vi "RT Main - 9035.vi"() -> ()   [LabVIEW 2017]
uses:
  Controls/Logging Settings.ctl
  Support Vis/Message Queue/Message Cluster.ctl
  Controls/Manual Control.ctl
  Controls/Manual Control FPGA.ctl
  Controls/Logging Settings FPGA.ctl
  Globals/Host/Global - Configuration Options.vi
  Globals/RT/Globals - RT Stream.vi
  <vilib>/Utility/error.llb/Error Cluster From Error Code.vi
  <vilib>/rvi/errors/niLvFpgaAdjustHostInterfaceError.vi
  Globals/RT/Global - Valves.vi
  <vilib>/rvi/interface/nirviReadWriteControl/nirviReadWriteControl.xnode
  Support Vis/Message Queue/Message Queue.lvlib
  NiFpgaLv.dll
  <vilib>/rvi/interface/Simulation/niFpgaSimulationCallBeginRW.vi
panel:
  out "Ready to log":bool
  out "Logging Information":T1={"Logging Channels"={"TC Logging"={"TC 0"=FALSE, "TC 1"=FALSE, "TC 2"=FALSE, "TC 3"=FALSE, "TC 4"=FALSE, "TC 5"=FALSE, "TC 6"=FALSE, "TC 7"=FALSE, "TC 8"=FALSE, "TC 9"=FALSE, "TC 10"=FALSE, "TC 11"=FALSE, "TC 12"=FALSE, "TC 13"=FALSE, "TC 14"=FALSE, "TC 15"=FALSE}, "PS Logging"={"PS 0"=FALSE, "PS 1"=FALSE, "PS 2"=FALSE, "PS 3"=FALSE, "PS 4"=FALSE, "PS 5"=FALSE, "PS 6"=FALSE, "PS 7"=FALSE}, "LC Logging"={"LC 0"=FALSE, "LC 1"=FALSE, "LC 2"=FALSE, "LC 3"=FALSE}}, "TC Low Speed Logging [Hz]"=1, "TC High Speed Logging [Hz]"=1, "PS Low Speed Logging [Hz]"=1, "PS High Speed Logging [Hz]"=1, "LC Low Speed Logging [Hz]"=1, "LC High Speed Logging[Hz]"=1, "Valve Names"=[]}
  out "Logging":bool
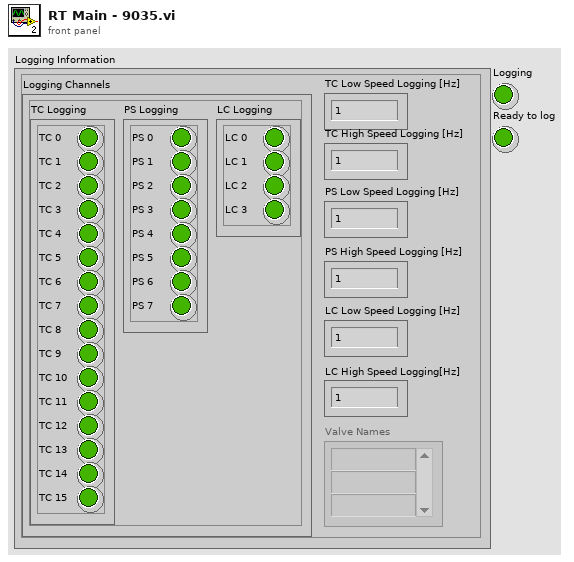
[diagram p1: front panel]
types:
  T1 = typedef "Logging Settings.ctl" = cluster{"Logging Channels":cluster{"TC Logging":cluster{"TC 0":bool, "TC 1":bool, "TC 2":bool, "TC 3":bool, "TC 4":bool, "TC 5":bool, "TC 6":bool, "TC 7":bool, "TC 8":bool, "TC 9":bool, "TC 10":bool, "TC 11":bool, "TC 12":bool, "TC 13":bool, "TC 14":bool, "TC 15":bool}, "PS Logging":cluster{"PS 0":bool, "PS 1":bool, "PS 2":bool, "PS 3":bool, "PS 4":bool, "PS 5":bool, "PS 6":bool, "PS 7":bool}, "LC Logging":cluster{"LC 0":bool, "LC 1":bool, "LC 2":bool, "LC 3":bool}}, "TC Low Speed Logging [Hz]":u32, "TC High Speed Logging [Hz]":u32, "PS Low Speed Logging [Hz]":u32, "PS High Speed Logging [Hz]":u32, "LC Low Speed Logging [Hz]":u32, "LC High Speed Logging[Hz]":u32, "Valve Names":string[]}
  T2 = typedef "Logging names.ctl" = cluster{"Keys":string[], "TC Names":string[], "PC Names":string[], "LC Names":string[], "Valve Names":string[]}
  T3 = cluster{"TC FIFO":refnum<k33>, "PS FIFO":refnum<k33>, "LC FIFO":refnum<k33>, "Valve FIFO":refnum<k33>}
  T4 = typedef "Message Queue.lvlib/All Real-Time Message Queues.ctl" = cluster{"Message Handler":refnum<queue>, "Acquisition and Logging":refnum<queue>}
  T5 = typedef "Message Queue.lvlib/Message Cluster.ctl" = cluster{"Message":string, "Message Data":variant}
  T6 = typedef "Manual Control.ctl" = cluster{"Actuator Settings":cluster{"Actuator Name":string, "Unpowered State":i16, "Output Port":u32, "Emergency State":i16, "Blank Button":bool, "Open Time [ms]":i16, "Close Time [ms]":i16}[]}
  T7 = typedef "Manual Control FPGA.ctl" = cluster{"Unpowered State":u8, "Output Port":u8, "Emergency State":u8, "Blank Button":bool, "Open Time [ms]":fxp<+/-,18,18>, "Close Time [ms]":fxp<+/-,18,18>, "Active":bool}[]
  T8 = typedef "Logging Settings FPGA.ctl" = cluster{"TC Low Speed Logging":u32, "TC  High Speed Logging":u32, "PS Low Speed Logging":u32, "PS  High Speed Logging":u32, "LC Low Speed Logging":u32, "LC  High Speed Logging":u32}
  T9 = enum16{"Manual", "Standby", "Automated Sequence", "Automated Sequence End", "Emergency"}
  T10 = cluster{"Actuator Name":string, "Unpowered State":i16, "Output Port":u32, "Emergency State":i16, "Blank Button":bool, "Open Time [ms]":i16, "Close Time [ms]":i16}[]
  T11 = cluster{"Unpowered State":u8, "Output Port":u8, "Emergency State":u8, "Blank Button":bool, "Open Time [ms]":fxp<+/-,18,18>, "Close Time [ms]":fxp<+/-,18,18>, "Active":bool}
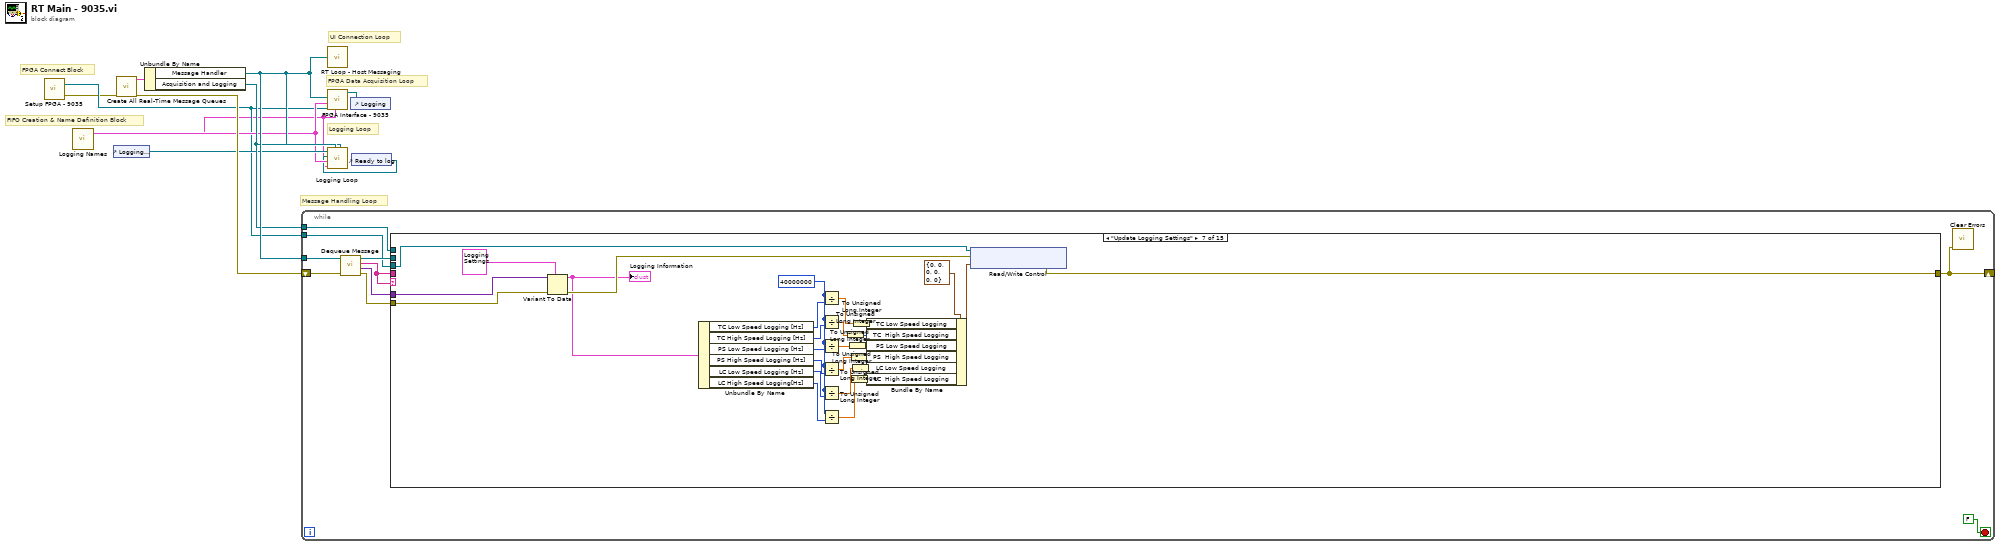
[diagram p0: block diagram]
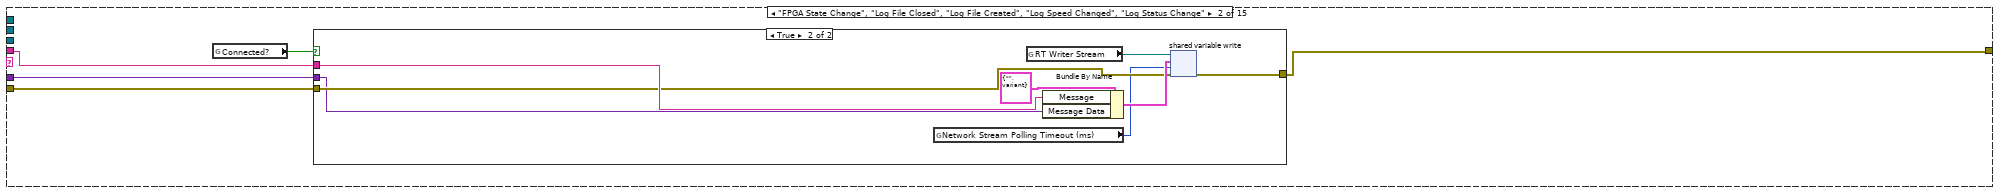
[diagram p3: hidden frame]
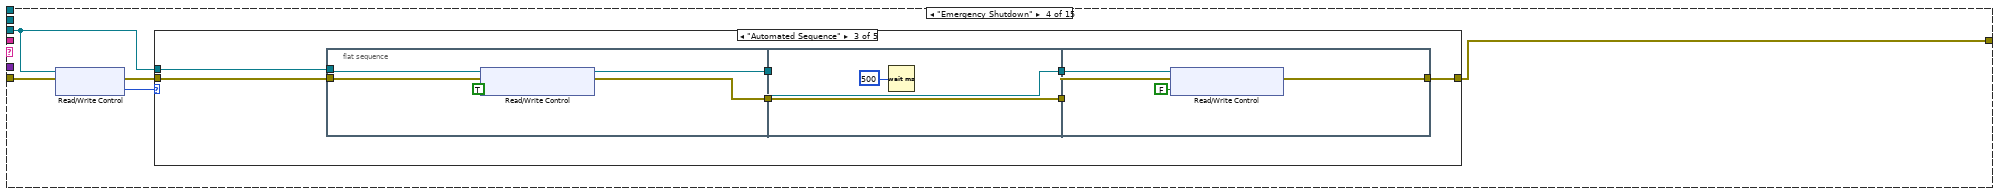
[diagram p6: hidden frame]
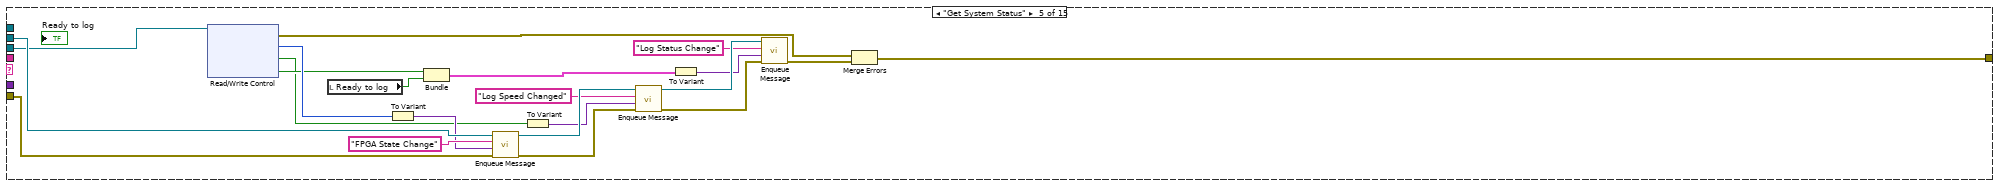
[diagram p11: hidden frame]
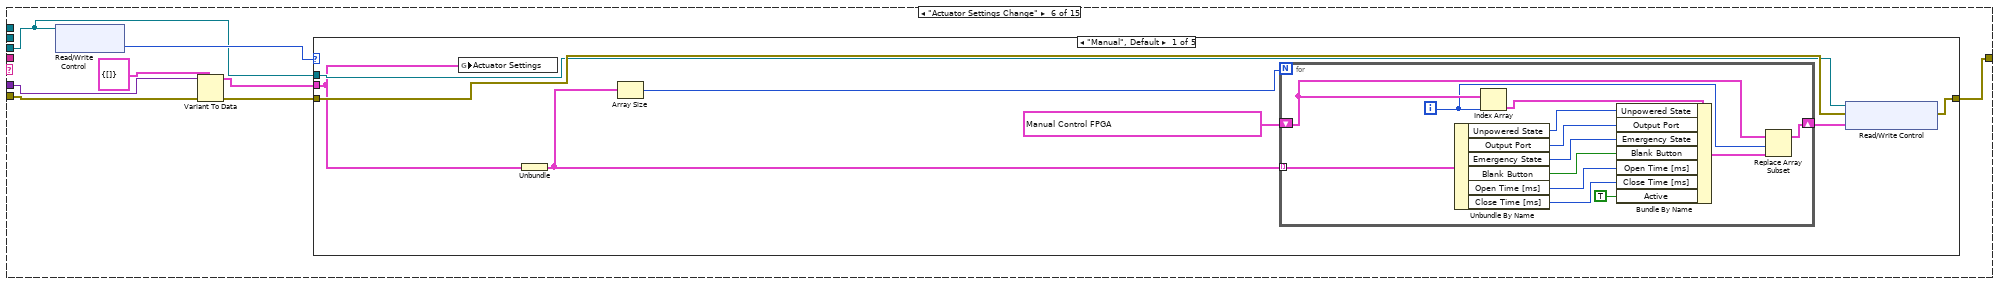
[diagram p12: hidden frame]
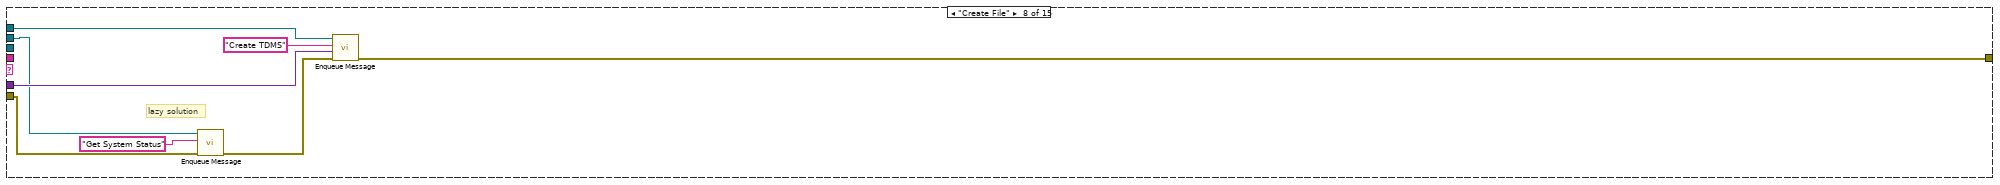
[diagram p17: hidden frame]
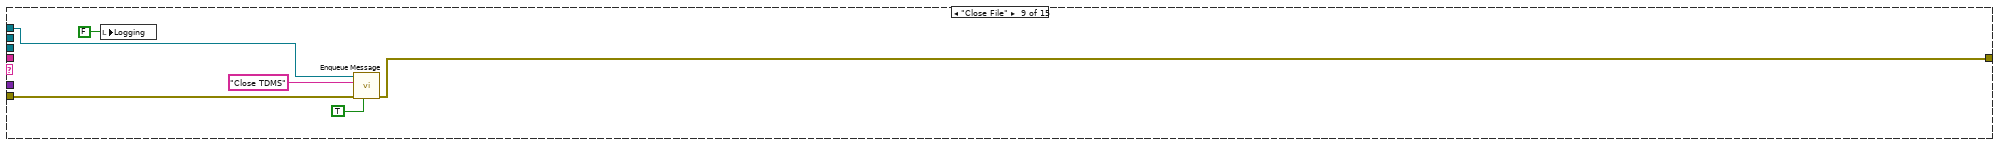
[diagram p18: hidden frame]
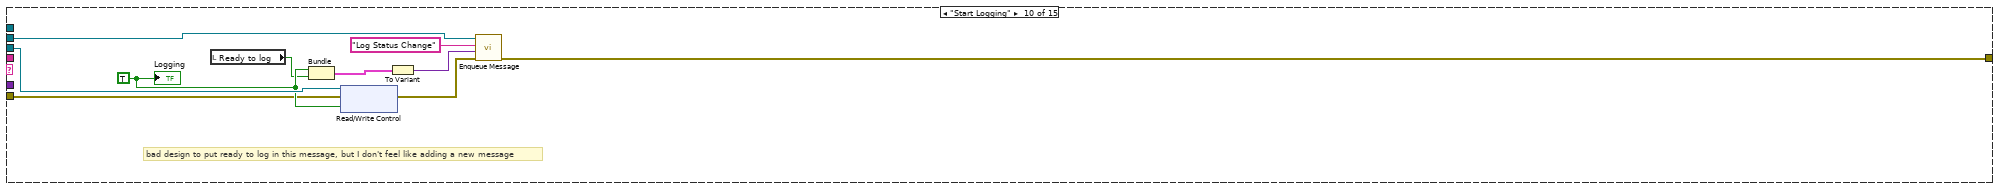
[diagram p19: hidden frame]
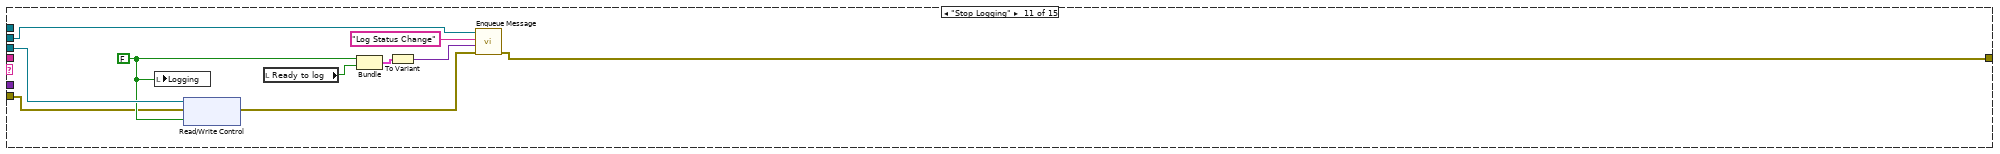
[diagram p20: hidden frame]
diagram:
  # "FPGA Connect Block"
  # "FIFO Creation & Name Definition Block"
  # "Message Handling Loop"
  # "Logging Loop"
  # "FPGA Data Acquisition Loop"
  # "UI Connection Loop"
  n1 = call "Setup FPGA - 9035.vi"() -> ("Error Out"=w2:errorcluster, "FPGA VI Reference Out"=w3:refnum<k20>)  [unwired: 2 in]
  n2 = call "Logging Names.vi"() -> ("Name Cluster"=w5:T2, "FIFO Cluster"=w1:T3)  [unwired: 3 in, 1 out]
  n3 = control-ref of="Logging Information"() -> (w6:refnum<vi>)
  n4 = call "Create All Real-Time Message Queues.vi"("error in (no error)"=w2) -> ("error out"=w10:errorcluster, "Message Queues out"=w11:T4)  [unwired: 9 in]
  n5 = Unbundle By Name(w11) -> ("Message Handler"=w8:refnum<queue>, "Acquisition and Logging"=w7:refnum<queue>)
  n6 = while {
    tunnel: w8 -> [w21]
    shift-right: [w12] -> _
    shift-left: w10 -> [w16]
    tunnel: w3 -> [w14]
    tunnel: w7 -> [w15]
    stop <- FALSE stop-if-true
    n7 = call "Dequeue Message.vi"("error in (no error)"=w16, "Message Queue"=w21) -> ("error out"=w13:errorcluster, "Message Data"=w19:variant, "Message"=w18:string, "dup Message Queue"=w20:refnum<queue>)  [unwired: 6 in]
    n8 = case shown="\"Update Logging Settings\"" w18 {
      tunnel: w20 -> [_ _ _ _ w86 _ _ w150 _ w170 w179 w186 _ _ _]
      tunnel: w18 -> [_ w27 _ _ _ _ _ _ _ _ _ _ _ _ _]
      tunnel: w19 -> [_ w25 _ _ _ w93 w147 w152 _ _ _ _ _ _ _]
      tunnel: [w22 w26 w37 w39 w81 w88 w143 w153 w158 w165 w175 w185 w199 w206 w224] -> w12
      tunnel: w14 -> [_ _ _ w41 w83 w90 w145 _ _ w171 w181 w191 w200 w205 _]
      tunnel: w15 -> [_ _ _ _ _ _ _ w155 w160 _ _ _ _ _ _]
      tunnel: w13 -> [w22 w23 w37 w38 w68 w87 w139 w149 w161 w164 w174 w182 w198 w211 w224]
      frame "Initialize" {
      }
      frame "FPGA State Change", "Log File Closed", "Log File Created", "Log Speed Changed", "Log Status Change" {
        n9 = global read "Global - Configuration Options.vi" "Connected?"() -> (w24:bool)
        n10 = case shown="True" w24 {
          tunnel: w27 -> [_ w36]
          tunnel: w23 -> [w28 w33]
          tunnel: [w28 w30] -> w26
          tunnel: w25 -> [_ w29]
          frame False {
          }
          frame True {
            n11 = global read "Global - Configuration Options.vi" "Network Stream Polling Timeout (ms)"() -> (w32:i32)
            n12 = global read "Globals - RT Stream.vi" "RT Writer Stream"() -> (w31:refnum<k21>)
            n13 = Bundle By Name(cluster=T5 {"Message"="", "Message Data"=variant} ("Message Cluster"), "Message"=w36, "Message Data"=w29) -> (w35:T5)
            n14 = shared-variable-write(w31, w33, w35, w32) -> (w30:errorcluster)  [unwired: 2 out]
          }
        }
      }
      frame "--------------" {
      }
      frame "Emergency Shutdown" {
        n15 = xnode "Read/Write Control"("FPGA VI Reference In"=w41, "error in"=w38) -> ("error out"=w40:errorcluster, "FPGA States"=w42:T9)  [unwired: 1 out]
        n16 = case shown="\"Automated Sequence\"" w42 {
          tunnel: w41 -> [_ _ w51 _ _]
          tunnel: w40 -> [w43 w44 w50 w64 w65]
          tunnel: [w43 w44 w45 w64 w65] -> w39
          frame "Manual", Default {
          }
          frame "Standby" {
          }
          frame "Automated Sequence" {
            n17 = flat-sequence {
              tunnel: w51 -> [w56]
              tunnel: w50 -> [w54]
              tunnel: [w53] -> w49
              tunnel: [w52] -> w48
              tunnel: w49 -> [w59]
              tunnel: w48 -> [w58]
              tunnel: [w59] -> w47
              tunnel: [w58] -> w46
              tunnel: w47 -> [w62]
              tunnel: w46 -> [w63]
              tunnel: [w60] -> w45
              frame #0 {
                n18 = xnode "Read/Write Control"("FPGA VI Reference In"=w56, "error in"=w54, "Emergency Shutdown"=TRUE) -> ("FPGA VI Reference Out"=w52:refnum<k20>, "error out"=w53:errorcluster)
              }
              frame #1 {
                n19 = Wait (ms)(milliseconds to wait=u32 500) -> ()  [unwired: 1 out]
              }
              frame #2 {
                n20 = xnode "Read/Write Control"("FPGA VI Reference In"=w63, "error in"=w62, "Emergency Shutdown"=FALSE) -> ("error out"=w60:errorcluster)  [unwired: 1 out]
              }
            }
          }
          frame "Automated Sequence End" {
          }
          frame "Emergency" {
          }
        }
      }
      frame "Get System Status" {
        n21 = xnode "Read/Write Control"("FPGA VI Reference In"=w83) -> ("error out"=w80:errorcluster, "FPGA States"=w82:T9, "High Speed?"=w69:bool, "Logging?"=w70:bool)  [unwired: 1 in, 1 out]
        n22 = local read "Ready to log"() -> (w66:bool)
        n23 = To Variant(anything=w82) -> (Variant=w84:variant)
        n24 = Bundle("Logging?"=w70, "Ready to log"=w66) -> (w67:cluster{"Logging?":bool, "Ready to log":bool})  [unwired: 1 in]
        n25 = call "Enqueue Message.vi"("error in (no error)"=w68, "Message Data"=w84, "Message"="FPGA State Change", "Message Queue"=w86) -> ("error out"=w79:errorcluster, "dup Message Queue"=w78:refnum<queue>)  [unwired: 6 in]
        n26 = To Variant(anything=w69) -> (Variant=w76:variant)
        n27 = call "Enqueue Message.vi"("error in (no error)"=w79, "Message Data"=w76, "Message"="Log Speed Changed", "Message Queue"=w78) -> ("error out"=w75:errorcluster, "dup Message Queue"=w74:refnum<queue>)  [unwired: 6 in]
        n28 = To Variant(anything=w67) -> (Variant=w71:variant)
        n29 = call "Enqueue Message.vi"("error in (no error)"=w75, "Message Data"=w71, "Message"="Log Status Change", "Message Queue"=w74) -> ("error out"=w73:errorcluster)  [unwired: 6 in, 1 out]
        n30 = Merge Errors(w80, w73) -> (w81:errorcluster)
      }
      frame "Actuator Settings Change" {
        n31 = xnode "Read/Write Control"("FPGA VI Reference In"=w90) -> ("FPGA States"=w94:T9)  [unwired: 1 in, 2 out]
        n32 = Variant To Data(error in=w87, type=T6 {"Actuator Settings"=[]} ("Actuator Settings"), Variant=w93) -> (data=w92:T6, error out=w91:errorcluster)
        n33 = case shown="\"Manual\", Default" w94 {
          tunnel: w90 -> [w100 _ _ _ _]
          tunnel: w92 -> [w97 _ _ _ _]
          tunnel: w91 -> [w102 w116 w117 w118 w119]
          tunnel: [w101 w116 w117 w118 w119] -> w88
          frame "Manual", Default {
            n34 = global write "Global - Valves.vi" "Actuator Settings"(w97) -> ()
            n35 = Unbundle(w97) -> ("Actuator Settings"=w98:T10)
            n36 = Array Size(array=w98) -> (size(s)=w99:i32)
            n37 = for {
              N: w99 -> [_]
              tunnel: w98 -> [w115] mode=indexing
              shift-right: [w114] -> w95
              shift-left: T7 [{"Unpowered State"=0, "Output Port"=0, "Emergency State"=0, "Blank Button"=FALSE, "Open Time [ms]"=0.0, "Close Time [ms]"=0.0, "Active"=FALSE}, {"Unpowered State"=0, "Output Port"=0, "Emergency State"=0, "Blank Button"=FALSE, "Open Time [ms]"=0.0, "Close Time [ms]"=0.0, "Active"=FALSE}, {"Unpowered State"=0, "Output Port"=0, "Emergency State"=0, "Blank Button"=FALSE, "Open Time [ms]"=0.0, "Close Time [ms]"=0.0, "Active"=FALSE}, {"Unpowered State"=0, "Output Port"=0, "Emergency State"=0, "Blank Button"=FALSE, "Open Time [ms]"=0.0, "Close Time [ms]"=0.0, "Active"=FALSE}, {"Unpowered State"=0, "Output Port"=0, "Emergency State"=0, "Blank Button"=FALSE, "Open Time [ms]"=0.0, "Close Time [ms]"=0.0, "Active"=FALSE}, {"Unpowered State"=0, "Output Port"=0, "Emergency State"=0, "Blank Button"=FALSE, "Open Time [ms]"=0.0, "Close Time [ms]"=0.0, "Active"=FALSE}, {"Unpowered State"=0, "Output Port"=0, "Emergency State"=0, "Blank Button"=FALSE, "Open Time [ms]"=0.0, "Close Time [ms]"=0.0, "Active"=FALSE}, {"Unpowered State"=0, "Output Port"=0, "Emergency State"=0, "Blank Button"=FALSE, "Open Time [ms]"=0.0, "Close Time [ms]"=0.0, "Active"=FALSE}, {"Unpowered State"=0, "Output Port"=0, "Emergency State"=0, "Blank Button"=FALSE, "Open Time [ms]"=0.0, "Close Time [ms]"=0.0, "Active"=FALSE}, {"Unpowered State"=0, "Output Port"=0, "Emergency State"=0, "Blank Button"=FALSE, "Open Time [ms]"=0.0, "Close Time [ms]"=0.0, "Active"=FALSE}, {"Unpowered State"=0, "Output Port"=0, "Emergency State"=0, "Blank Button"=FALSE, "Open Time [ms]"=0.0, "Close Time [ms]"=0.0, "Active"=FALSE}, {"Unpowered State"=0, "Output Port"=0, "Emergency State"=0, "Blank Button"=FALSE, "Open Time [ms]"=0.0, "Close Time [ms]"=0.0, "Active"=FALSE}, {"Unpowered State"=0, "Output Port"=0, "Emergency State"=0, "Blank Button"=FALSE, "Open Time [ms]"=0.0, "Close Time [ms]"=0.0, "Active"=FALSE}, {"Unpowered State"=0, "Output Port"=0, "Emergency State"=0, "Blank Button"=FALSE, "Open Time [ms]"=0.0, "Close Time [ms]"=0.0, "Active"=FALSE}, {"Unpowered State"=0, "Output Port"=0, "Emergency State"=0, "Blank Button"=FALSE, "Open Time [ms]"=0.0, "Close Time [ms]"=0.0, "Active"=FALSE}] ("Actuator Settings 2") -> [w113]
              i -> [w110]
              n38 = Unbundle By Name(w115) -> ("Unpowered State"=w103:i16, "Output Port"=w104:u32, "Emergency State"=w105:i16, "Blank Button"=w106:bool, "Open Time [ms]"=w107:i16, "Close Time [ms]"=w108:i16)
              n39 = Index Array(array=w113, index=w110) -> (element=w112:T11)
              n40 = Bundle By Name(cluster=w112, "Unpowered State"=w103, "Output Port"=w104, "Emergency State"=w105, "Blank Button"=w106, "Open Time [ms]"=w107, "Close Time [ms]"=w108, "Active"=TRUE) -> (w111:T11)
              n41 = Replace Array Subset(array=w113, new element=w111, index=w110) -> (w114:T7)
            }
            n42 = xnode "Read/Write Control"("FPGA VI Reference In"=w100, "error in"=w102, "Actuator Settings"=w95) -> ("error out"=w101:errorcluster)  [unwired: 1 out]
          }
          frame "Standby" {
          }
          frame "Automated Sequence" {
          }
          frame "Automated Sequence End" {
          }
          frame "Emergency" {
          }
        }
      }
      frame "Update Logging Settings" {
        w138 = 40000000
        n43 = Variant To Data(error in=w139, type=T1 {"Logging Channels"={"TC Logging"={"TC 0"=FALSE, "TC 1"=FALSE, "TC 2"=FALSE, "TC 3"=FALSE, "TC 4"=FALSE, "TC 5"=FALSE, "TC 6"=FALSE, "TC 7"=FALSE, "TC 8"=FALSE, "TC 9"=FALSE, "TC 10"=FALSE, "TC 11"=FALSE, "TC 12"=FALSE, "TC 13"=FALSE, "TC 14"=FALSE, "TC 15"=FALSE}, "PS Logging"={"PS 0"=FALSE, "PS 1"=FALSE, "PS 2"=FALSE, "PS 3"=FALSE, "PS 4"=FALSE, "PS 5"=FALSE, "PS 6"=FALSE, "PS 7"=FALSE}, "LC Logging"={"LC 0"=FALSE, "LC 1"=FALSE, "LC 2"=FALSE, "LC 3"=FALSE}}, "TC Low Speed Logging [Hz]"=0, "TC High Speed Logging [Hz]"=0, "PS Low Speed Logging [Hz]"=0, "PS High Speed Logging [Hz]"=0, "LC Low Speed Logging [Hz]"=0, "LC High Speed Logging[Hz]"=0, "Valve Names"=[]} ("Cluster"), Variant=w147) -> (data=w142:T1, error out=w144:errorcluster)
        "Logging Information" <- w142
        n44 = Unbundle By Name(w142) -> ("TC Low Speed Logging [Hz]"=w137:u32, "TC High Speed Logging [Hz]"=w136:u32, "PS Low Speed Logging [Hz]"=w135:u32, "PS High Speed Logging [Hz]"=w134:u32, "LC Low Speed Logging [Hz]"=w133:u32, "LC High Speed Logging[Hz]"=w132:u32)
        n45 = Divide(x=w138, y=w137) -> (x/y=w126:dbl)
        n46 = Divide(x=w138, y=w136) -> (x/y=w127:dbl)
        n47 = Divide(x=w138, y=w135) -> (x/y=w128:dbl)
        n48 = Divide(x=w138, y=w134) -> (x/y=w129:dbl)
        n49 = Divide(x=w138, y=w133) -> (x/y=w130:dbl)
        n50 = Divide(x=w138, y=w132) -> (x/y=w131:dbl)
        n51 = To Unsigned Long Integer(number=w127) -> (unsigned 32bit integer=w124:u32)
        n52 = To Unsigned Long Integer(number=w128) -> (unsigned 32bit integer=w123:u32)
        n53 = To Unsigned Long Integer(number=w129) -> (unsigned 32bit integer=w122:u32)
        n54 = To Unsigned Long Integer(number=w131) -> (unsigned 32bit integer=w120:u32)
        n55 = To Unsigned Long Integer(number=w130) -> (unsigned 32bit integer=w121:u32)
        n56 = To Unsigned Long Integer(number=w126) -> (unsigned 32bit integer=w125:u32)
        n57 = Bundle By Name(cluster=T8 {"TC Low Speed Logging"=0, "TC  High Speed Logging"=0, "PS Low Speed Logging"=0, "PS  High Speed Logging"=0, "LC Low Speed Logging"=0, "LC  High Speed Logging"=0} ("Cluster"), "TC Low Speed Logging"=w125, "TC  High Speed Logging"=w124, "PS Low Speed Logging"=w123, "PS  High Speed Logging"=w122, "LC Low Speed Logging"=w121, "LC  High Speed Logging"=w120) -> (w140:T8)
        n58 = xnode "Read/Write Control"("FPGA VI Reference In"=w145, "error in"=w144, "Logging Settings [Ticks]"=w140) -> ("error out"=w143:errorcluster)  [unwired: 1 out]
      }
      frame "Create File" {
        # "lazy solution"
        n59 = call "Enqueue Message.vi"("error in (no error)"=w149, "Message"="Get System Status", "Message Queue"=w150) -> ("error out"=w148:errorcluster)  [unwired: 7 in, 1 out]
        n60 = call "Enqueue Message.vi"("error in (no error)"=w148, "Message Data"=w152, "Message"="Create TDMS", "Message Queue"=w155) -> ("error out"=w153:errorcluster)  [unwired: 6 in, 1 out]
      }
      frame "Close File" {
        n61 = local write "Logging"(FALSE ("Logging")) -> ()
        n62 = call "Enqueue Message.vi"("Priority Message? (F)"=TRUE, "error in (no error)"=w161, "Message"="Close TDMS", "Message Queue"=w160) -> ("error out"=w158:errorcluster)  [unwired: 6 in, 1 out]
      }
      frame "Start Logging" {
        w166 = TRUE ("Logging")
        # "bad design to put ready to log in this message, but I don't feel like adding a new message"
        n63 = local read "Ready to log"() -> (w162:bool)
        n64 = Bundle("Logging"=w166, "Ready to log"=w162) -> (w163:cluster{"Logging":bool, "Ready to log":bool})  [unwired: 1 in]
        n65 = xnode "Read/Write Control"("FPGA VI Reference In"=w171, "error in"=w164, "Logging?"=w166) -> ("error out"=w168:errorcluster)  [unwired: 1 out]
        n66 = To Variant(anything=w163) -> (Variant=w167:variant)
        n67 = call "Enqueue Message.vi"("error in (no error)"=w168, "Message Data"=w167, "Message"="Log Status Change", "Message Queue"=w170) -> ("error out"=w165:errorcluster)  [unwired: 6 in, 1 out]
        "Logging" <- w166
      }
      frame "Stop Logging" {
        w176 = FALSE ("Logging")
        n68 = local write "Logging"(w176) -> ()
        n69 = xnode "Read/Write Control"("FPGA VI Reference In"=w181, "error in"=w174, "Logging?"=w176) -> ("error out"=w180:errorcluster)  [unwired: 1 out]
        n70 = local read "Ready to log"() -> (w172:bool)
        n71 = Bundle("Logging"=w176, "Ready to log"=w172) -> (w173:cluster{"Logging":bool, "Ready to log":bool})  [unwired: 1 in]
        n72 = To Variant(anything=w173) -> (Variant=w177:variant)
        n73 = call "Enqueue Message.vi"("error in (no error)"=w180, "Message Data"=w177, "Message"="Log Status Change", "Message Queue"=w179) -> ("error out"=w175:errorcluster)  [unwired: 6 in, 1 out]
      }
      frame "Toggle Logging Mode" {
        n74 = xnode "Read/Write Control"("FPGA VI Reference In"=w191, "error in"=w182) -> ("FPGA VI Reference Out"=w190:refnum<k20>, "error out"=w188:errorcluster, "High Speed?"=w189:bool)
        n75 = Not(x=w189) -> (.not. x?=w183:bool)
        n76 = xnode "Read/Write Control"("FPGA VI Reference In"=w190, "error in"=w188, "High Speed?"=w183) -> ("error out"=w187:errorcluster)  [unwired: 1 out]
        n77 = case shown="No Error" w187 {
          tunnel: w186 -> [w196 _]
          tunnel: [w194 errorcluster {"status"=FALSE, "code"=0, "source"=""} ("error out")] -> w184
          tunnel: w183 -> [w192 _]
          frame No Error {
            n78 = To Variant(anything=w192) -> (Variant=w193:variant)
            n79 = call "Enqueue Message.vi"("Message Data"=w193, "Message"="Log Speed Changed", "Message Queue"=w196) -> ("error out"=w194:errorcluster)  [unwired: 7 in, 1 out]
          }
          frame Error {
          }
        }
        n80 = Merge Errors(w184, w187) -> (w185:errorcluster)
      }
      frame "Toggle Manual Mode" {
        n81 = xnode "Read/Write Control"("FPGA VI Reference In"=w200, "error in"=w198) -> ("FPGA VI Reference Out"=w204:refnum<k20>, "error out"=w202:errorcluster, "Manual Mode"=w203:bool)
        n82 = Not(x=w203) -> (.not. x?=w201:bool)
        n83 = xnode "Read/Write Control"("FPGA VI Reference In"=w204, "error in"=w202, "Manual Mode"=w201) -> ("error out"=w199:errorcluster)  [unwired: 1 out]
      }
      frame "Start AC" {
        n84 = flat-sequence {
          tunnel: w205 -> [w216]
          tunnel: w211 -> [w215]
          tunnel: [w213] -> w209
          tunnel: [w212] -> w207
          tunnel: [w218] -> w210
          tunnel: w209 -> [w218]
          tunnel: [w217] -> w208
          tunnel: w207 -> [w217]
          tunnel: w210 -> [w223]
          tunnel: w208 -> [w222]
          tunnel: [w220] -> w206
          frame #0 {
            n85 = xnode "Read/Write Control"("FPGA VI Reference In"=w216, "error in"=w215, "Start Automated Sequence"=TRUE) -> ("FPGA VI Reference Out"=w213:refnum<k20>, "error out"=w212:errorcluster)
          }
          frame #1 {
            n86 = Wait (ms)(milliseconds to wait=u32 50) -> ()  [unwired: 1 out]
          }
          frame #2 {
            n87 = xnode "Read/Write Control"("FPGA VI Reference In"=w223, "error in"=w222, "Start Automated Sequence"=FALSE) -> ("error out"=w220:errorcluster)  [unwired: 1 out]
          }
        }
      }
      frame Default {
      }
    }
    n88 = call <vilib>:"Clear Errors.vi"("error in (no error)"=w12) -> ()  [unwired: 5 in, 2 out]
  }
  n89 = call "RT Loop - Host Messaging.vi"("Message Queue"=w8) -> ()
  n90 = control-ref of="Logging"() -> (w9:refnum<vi>)
  n91 = call "FPGA Interface - 9035.vi"("FIFO Cluster"=w1, "FPGA VI Reference Out"=w3, "Name Cluster"=w5, "RT Main Message Handler"=w8, "Logging?"=w9) -> ()  [unwired: 7 in]
  n92 = control-ref of="Ready to log"() -> (w4:refnum<vi>)
  n93 = call "Logging Loop.vi"("Acquisition and Logging"=w7, "Message Handler"=w8, "FIFO Cluster"=w1, "Name Cluster"=w5, "Ready to log"=w4, "Logging Cluster"=w6) -> ()  [unwired: 6 in]
